vi "PXIe-4468_SineGenerator.vi"() -> ()   [LabVIEW 2025]
uses:
  <vilib>/DAQmx/create/channels.llb/DAQmx Create Channel (AO-Voltage-Basic).vi
panel:
  in  "Physical Channel(s)":tag
  out "error out":errorcluster
  in  "error in":errorcluster
  in  "Stop Button":bool
  in  "Start Button":bool
  in  "Amplitude (V Peak)":dbl format="%#_2f"
  in  "Device Max Sample Rate (S/s)":dbl
  out "Samples Per Cycle (N)":dbl
  out "Computed Sample Rate (S/s)":i32
  in  "Frequency (Hz)":u16(ring) items=["50", "60", "120", "8192", "29430"]
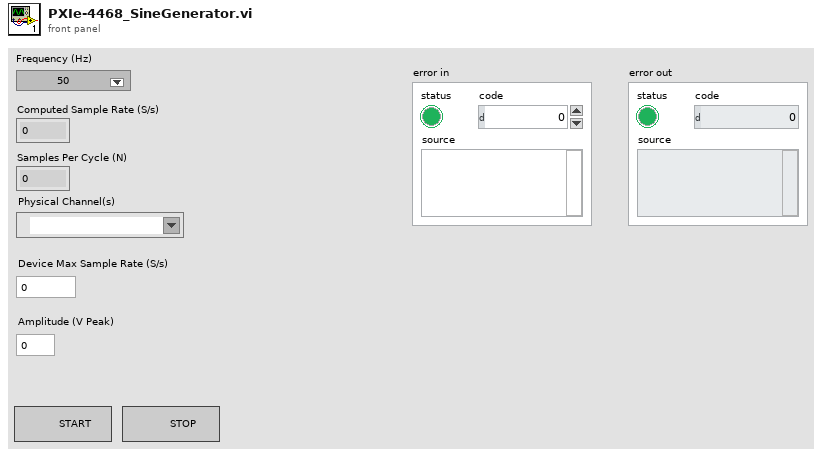
[diagram p1: front panel]
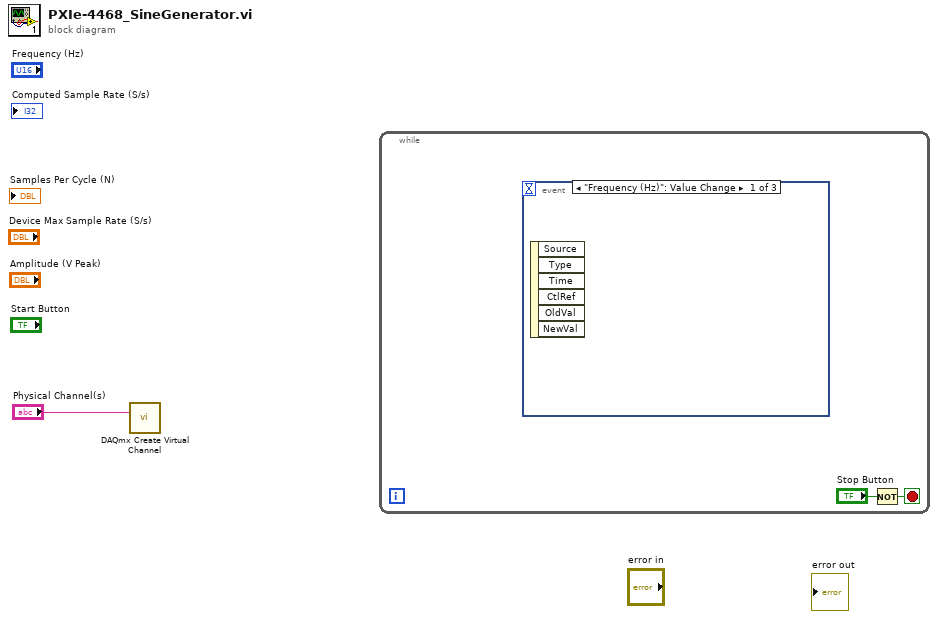
[diagram p0: block diagram]
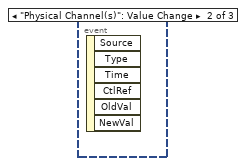
[diagram p2: hidden frame]
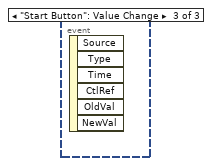
[diagram p3: hidden frame]
diagram:
  n1 = call-poly <vilib>:"DAQmx Create Virtual Channel.vi"("physical channels"="Physical Channel(s)") -> ()  [unwired: 13 in, 2 out]
  n2 = while {
    stop <- w2 stop-if-true
    n3 = event shown="[0] \"Frequency (Hz)\": Value Change" {
      selector: _ -> [_ _ _]
      dyn-events: _ -> [_ _ _]
      timeout: _ -> [_ _ _]
      event "Frequency (Hz)": Value Change {
        n4 = event-data() -> ()  [unwired: 1 in, 6 out]
      }
      event "Physical Channel(s)": Value Change {
        n5 = event-data() -> ()  [unwired: 1 in, 6 out]
      }
      event "Start Button": Value Change {
        n6 = event-data() -> ()  [unwired: 1 in, 6 out]
      }
    }
    n7 = Not(x="Stop Button") -> (.not. x?=w2:bool)
  }
